vi "Strip Quotes and Unescape.vi"(8 "error in (no error)":errorcluster, 11 "String":string) -> (0 "error out":errorcluster, 3 "result string":string)   [LabVIEW 2013, in "JSONtext support.lvlib"]
uses:
  JSONtext support.lvlib
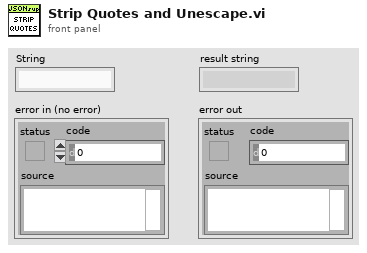
[diagram p1: front panel]
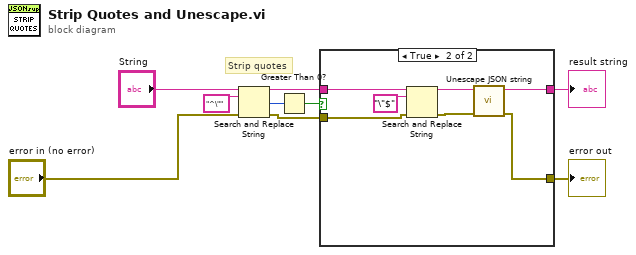
[diagram p0: block diagram]
diagram:
  # "Strip quotes"
  n1 = Search and Replace String(input string="String", search string="^\"", error in="error in (no error)") -> (result string=w5:string, number of replacements=w2:i32, error out=w8:errorcluster)  [unwired: 5 in, 1 out]
  n2 = Greater Than 0?(x=w2) -> (x > 0?=w1:bool)
  n3 = case shown="True" w1 {
    tunnel: [w10 w12] -> w9
    tunnel: w8 -> [w10 w18]
    tunnel: [w11 w14] -> w6
    tunnel: w5 -> [w11 w17]
    frame False {
    }
    frame True {
      n4 = Search and Replace String(input string=w17, search string="\"$", error in=w18) -> (result string=w15:string, error out=w13:errorcluster)  [unwired: 5 in, 2 out]
      n5 = call "Unescape JSON string.vi"("error in (no error)"=w13, "Text (with JSON escapes)"=w15) -> ("error out"=w12:errorcluster, "Text (unescaped)"=w14:string)  [unwired: 8 in]
    }
  }
  "error out" <- w9
  "result string" <- w6
